vi "MasterStateController.vi"() -> (8 "Master State Out":T1(ring), 12 "Confirmed Master States":bool[](array[boolean]), 13 "Disallowed Master States":bool[](array[boolean]))   [LabVIEW 2020]
doc: "This is the master robot state controller. The master robot state can affect any of the subsystem state controllers."
uses:
  7917f586-2427-458d-9aab-c53b65a4f0cc.vi
  GlobalDriverStationData.vi
  GlobalDriverStationCommands.vi
  GlobalArm.vi
  GlobalGripper.vi
  GlobalPoseAndTargeting.vi
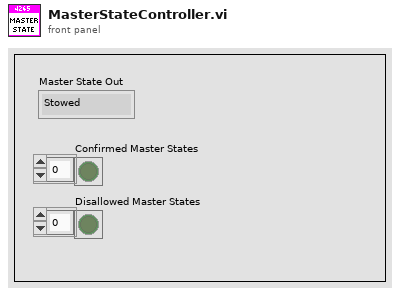
[diagram p1: front panel]
types:
  T1 = enum16{"Stowed", "Balancing", "Scoring", "Hoppering", "Ground", "Shelf"}
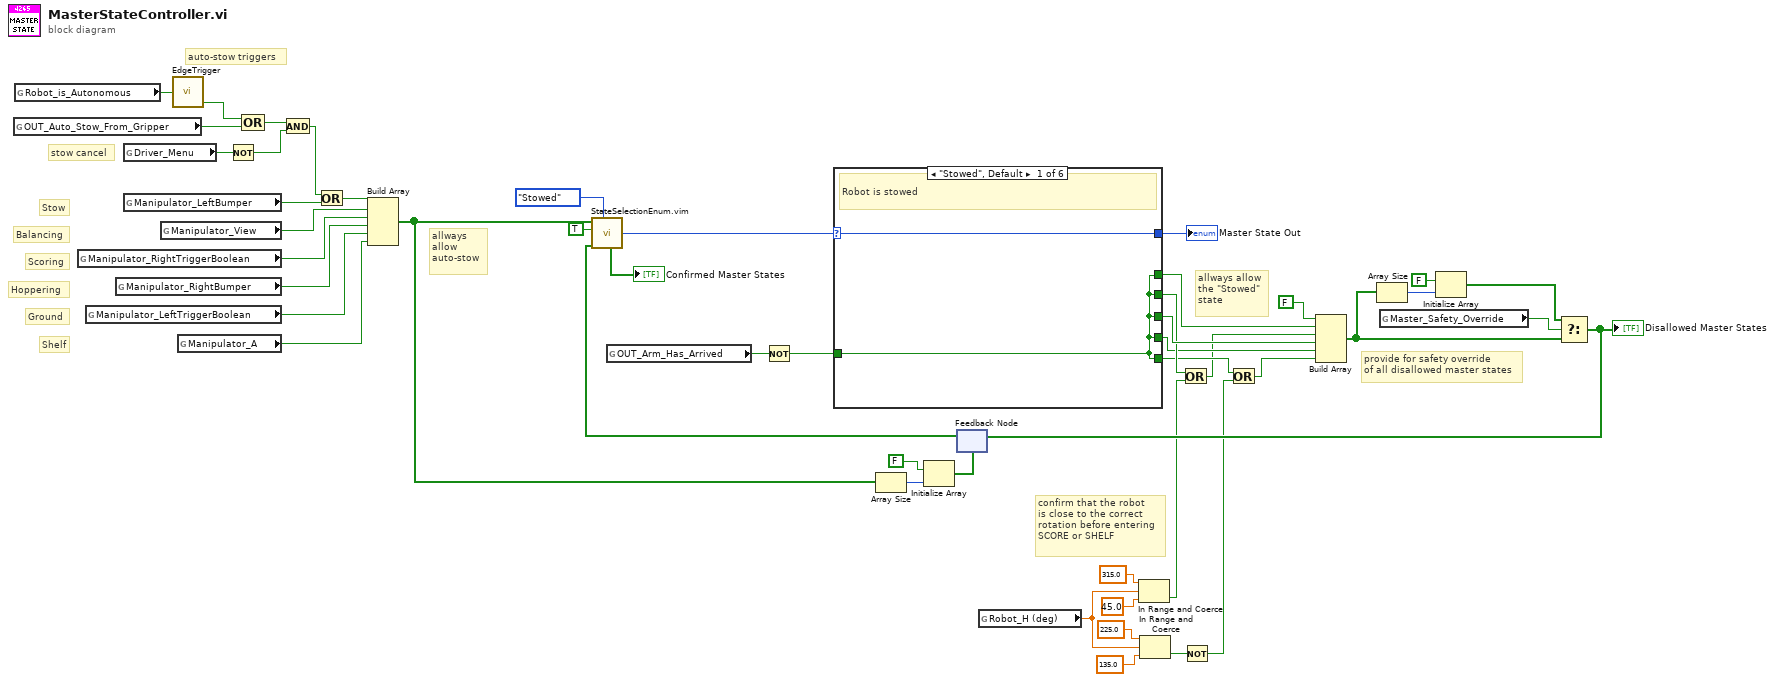
[diagram p0: block diagram]
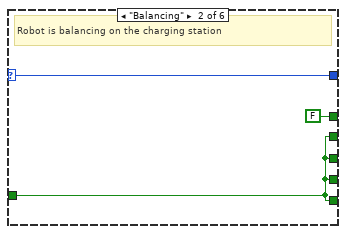
[diagram p2: hidden frame]
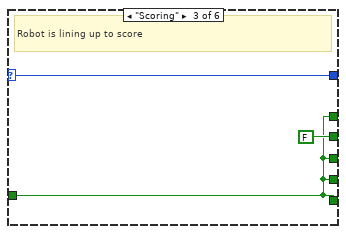
[diagram p3: hidden frame]
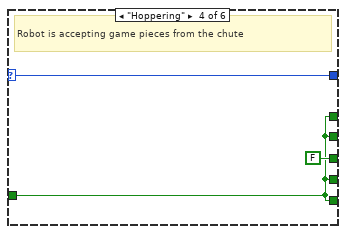
[diagram p4: hidden frame]
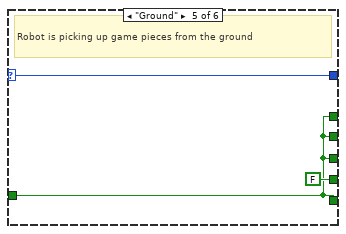
[diagram p5: hidden frame]
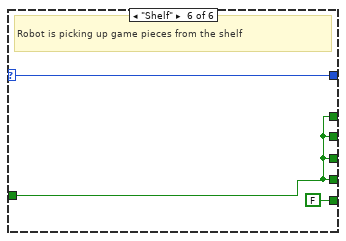
[diagram p6: hidden frame]
diagram:
  # "confirm that the robot\nis close to the correct\nrotation before entering\nSCORE or SHELF"
  # "allways allow\nthe \"Stowed\"\nstate"
  # "Shelf"
  # "Ground"
  # "Hoppering"
  # "Scoring"
  # "Balancing"
  # "Stow"
  # "stow cancel"
  # "allways\nallow\nauto-stow"
  # "auto-stow triggers"
  # "provide for safety override\nof all disallowed master states"
  n1 = global read "GlobalGripper.vi" "OUT_Auto_Stow_From_Gripper"() -> (w26:bool)
  n2 = global read "GlobalDriverStationData.vi" "Robot_is_Autonomous"() -> (w15:bool)
  n3 = global read "GlobalDriverStationCommands.vi" "Manipulator_RightTriggerBoolean"() -> (w32:bool)
  n4 = global read "GlobalDriverStationCommands.vi" "Manipulator_LeftTriggerBoolean"() -> (w30:bool)
  n5 = global read "GlobalDriverStationCommands.vi" "Manipulator_RightBumper"() -> (w31:bool)
  n6 = global read "GlobalDriverStationCommands.vi" "Driver_Menu"() -> (w20:bool)
  n7 = global read "GlobalDriverStationCommands.vi" "Manipulator_LeftBumper"() -> (w24:bool)
  n8 = global read "GlobalDriverStationCommands.vi" "Manipulator_View"() -> (w33:bool)
  n9 = call "EdgeTrigger.vi"("Input Signal"=w15) -> ("Falling Edge Trigger"=w16:bool)  [unwired: 2 out]
  n10 = global read "GlobalDriverStationCommands.vi" "Manipulator_A"() -> (w29:bool)
  n11 = Not(x=w20) -> (.not. x?=w19:bool)
  n12 = Compound Arithmetic op=OR(w16, w26) -> (w23:bool)
  n13 = And(x=w23, y=w19) -> (x .and. y?=w21:bool)
  n14 = Or(x=w21, y=w24) -> (x .or. y?=w22:bool)
  n15 = Build Array(w22, w33, w32, w31, w30, w29) -> (w28:bool[])
  n16 = global read "GlobalArm.vi" "OUT_Arm_Has_Arrived"() -> (w27:bool)
  n17 = Not(x=w27) -> (.not. x?=w18:bool)
  n18 = Array Size(array=w28) -> (size(s)=w36:i32)
  n19 = Initialize Array(FALSE, w36) -> (w34:bool[])
  n20 = feedback #1(w34) -> (w1:bool[])
  n21 = call "StateSelectionEnum.vim"("Enum Def"=T1."Stowed", "Disallowed States"=w1, "Enable Edge Trigger"=TRUE, "State Triggers"=w28) -> ("Selected State"=w25:T1, "Confirmed States"=→"Confirmed Master States":bool[])  [unwired: 1 in]
  n22 = case shown="\"Stowed\", Default" w25 {
    selector: w25 -> [w50 w53 w55 w58 w61 w64]
    tunnel: [w50 w53 w55 w58 w61 w64] -> w42
    tunnel: [w49 FALSE ("Normal") w54 w57 w60 w63] -> w43
    tunnel: [w49 w51 FALSE ("Normal") w57 w60 w63] -> w17
    tunnel: [w49 w51 w54 FALSE ("Normal") w60 w63] -> w41
    tunnel: [w49 w51 w54 w57 FALSE ("Normal") w63] -> w14
    tunnel: [w49 w51 w54 w57 w60 FALSE ("Normal")] -> w13
    tunnel: w18 -> [w49 w51 w54 w57 w60 w63]
    frame "Stowed", Default {
      # "Robot is stowed"
    }
    frame "Balancing" {
      # "Robot is balancing on the charging station"
    }
    frame "Scoring" {
      # "Robot is lining up to score"
    }
    frame "Hoppering" {
      # "Robot is accepting game pieces from the chute"
    }
    frame "Ground" {
      # "Robot is picking up game pieces from the ground"
    }
    frame "Shelf" {
      # "Robot is picking up game pieces from the shelf"
    }
  }
  "Master State Out" <- w42
  n23 = global read "GlobalPoseAndTargeting.vi" "Robot_H (deg)"() -> (w6:dbl)
  n24 = In Range and Coerce(upper limit=315.0, x=w6, lower limit=45.0) -> (In Range?=w9:bool)  [unwired: 1 out]
  n25 = In Range and Coerce(upper limit=225.0, x=w6, lower limit=135.0) -> (In Range?=w4:bool)  [unwired: 1 out]
  n26 = Or(x=w17, y=w9) -> (x .or. y?=w10:bool)
  n27 = Not(x=w4) -> (.not. x?=w3:bool)
  n28 = Or(x=w13, y=w3) -> (x .or. y?=w5:bool)
  n29 = Build Array(FALSE ("Normal"), w43, w10, w41, w14, w5) -> (w44:bool[])
  n30 = Array Size(array=w44) -> (size(s)=w47:i32)
  n31 = global read "GlobalDriverStationData.vi" "Master_Safety_Override"() -> (w48:bool)
  n32 = Initialize Array(FALSE ("element"), w47) -> (w45:bool[])
  n33 = Select(t=w45, s=w48, f=w44) -> (s? t:f=w37:bool[])
  "Disallowed Master States" <- w37
  n34 = feedback-in #1(w37) -> ()
